vi "FaceTracking.vi"(8 "error in (no error)":errorcluster, 10 "img in":T1, 11 "session in":refnum<k35>) -> (0 "error out":errorcluster, 1 "offset from center":dbl, 2 "img out":T1, 3 "session out":refnum<k35>)   [LabVIEW 2018]
uses:
  <vilib>/picture/picture.llb/imagedata.ctl
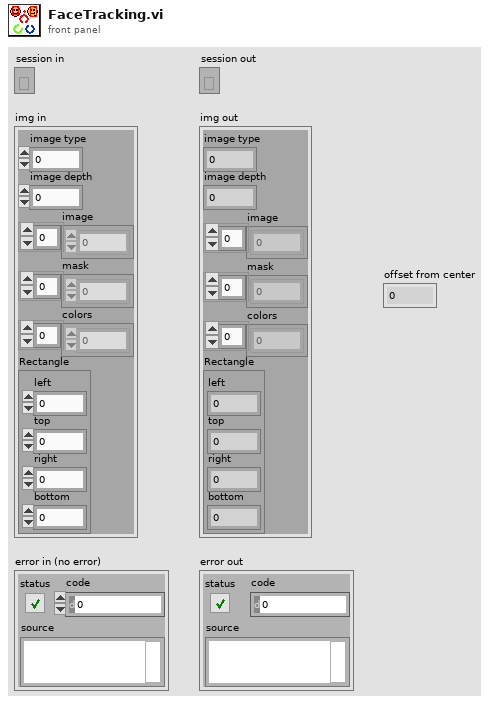
[diagram p1: front panel]
types:
  T1 = typedef "imagedata.ctl" = cluster{"image type":i32, "image depth":i32, "image":u8[], "mask":u8[], "colors":u32[], "Rectangle":cluster{"left":i16, "top":i16, "right":i16, "bottom":i16}}
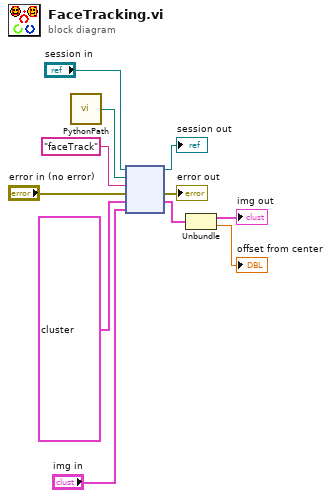
[diagram p0: block diagram]
diagram:
  n1 = call "PythonPath.vi"() -> ("path to .py"=w11:path)
  n2 = node("session in", w11, "faceTrack" ("function name"), "error in (no error)", cluster{"img data 2":T1, "image":dbl} {"img data 2"={"image type"=0, "image depth"=24, "image"=array[921600 elements], "mask"=[], "colors"=[], "Rectangle"={"left"=0, "top"=0, "right"=640, "bottom"=480}}, "image"=0.0} ("Cluster"), "img in") -> (→"session out":refnum<k35>, →"error out":errorcluster, w3:cluster{"img data 2":T1, "image":dbl})  [unwired: 1 in, 2 out]
  n3 = Unbundle(w3) -> ("img data 2"=→"img out":T1, "image"=→"offset from center":dbl)
